vi "Create_Experiment_Excel_Files.vi"(1 "error in":errorcluster, 2 "Folder path in":path, 3 "Data in":T1={"User Name"="", "Experiment Number"=0, "Start Time"=timestamp(0 s since 1904-01-01), "Data"=[], "Step Number"=1, "Step Instructions"="", "Diagnostics"={"Langmuir Probe"=FALSE, "Rogowski 1"=FALSE, "Rogowski 2"=FALSE, "Rogowski 3"=FALSE, "B-dot 1"=FALSE, "B-dot 2"=FALSE}, "Experiment Purpose"="", "Experiment State"=enum."Off", "Systems"={"Compressed Air"=FALSE, "T-20kV Power Switch"=FALSE, "T-Rectifier"=FALSE, "Engage Interlock"=FALSE, "Ventilator"=FALSE, "Magnetron"=FALSE, "H-20kV Power Switch"=FALSE, "H-Rectifier"=FALSE, "Main Water Pump"=FALSE, "WEGA Water Pump"=FALSE, "Gas Inlet Valves"=FALSE}, "Vacuum Pressure"=0.0, "Fieldpoints"={"System Boolean Fieldpoints"={"Compressed Air"="", "T-20kV Power Switch"="", "T-Rectifier"="", "Engage Interlock"="", "Ventilator"="", "Magnetron"="", "H-20kV Power Switch"="", "H-Rectifier"="", "Main Water Pump"="", "WEGA Water Pump"="", "Gas Inlet Valves"=""}, "Step Fieldpoints"={"Exhaust Ventillator"="", "Compressed Air"="", "Water Pressure"="", "Interlock"="", "Toroidal Power Supply 1"="", "Toroidal Power Supply 2"="", "Toroidal Rectifier"="", "Helical Power Supply"="", "Helical Rectifier"="", "6kW Magnetron Standby"="", "20kW Magnetron Standby"=""}}, "Pressure History"={"Seconds into Experiment"=[], "Pressure Data"=[]}, "Time Computer Control"=[], "Toroidal Voltage Computer Control"=[], "Helical Voltage Computer Control"=[], "Toroidal Current"=[], "Toroidal Voltage"=[], "Toroidal Current Set Point"=[], "Helical Current Set Point"=[], "Helical Voltage"=[], "Helical Current"=[], "Experiment Folder"=path "", "Run Another Shot?"=FALSE}) -> (0 "error out":errorcluster)   [LabVIEW 2017]
uses:
  Type_Defs/Data.ctl
  Type_Defs/Diagnostics.ctl
  Type_Defs/Systems.ctl
  <vilib>/express/express shared/transition.llb/Dynamic To Waveform Array.vi
  <vilib>/express/express signal manip/GetorSetDDTAttributes/Set DDT Attributes/SetT0.vi
  <vilib>/express/express shared/transition.llb/Waveform Array To Dynamic.vi
  <vilib>/express/express signal manip/GetorSetDDTAttributes/Set DDT Attributes/Set DDT Properties.xnode
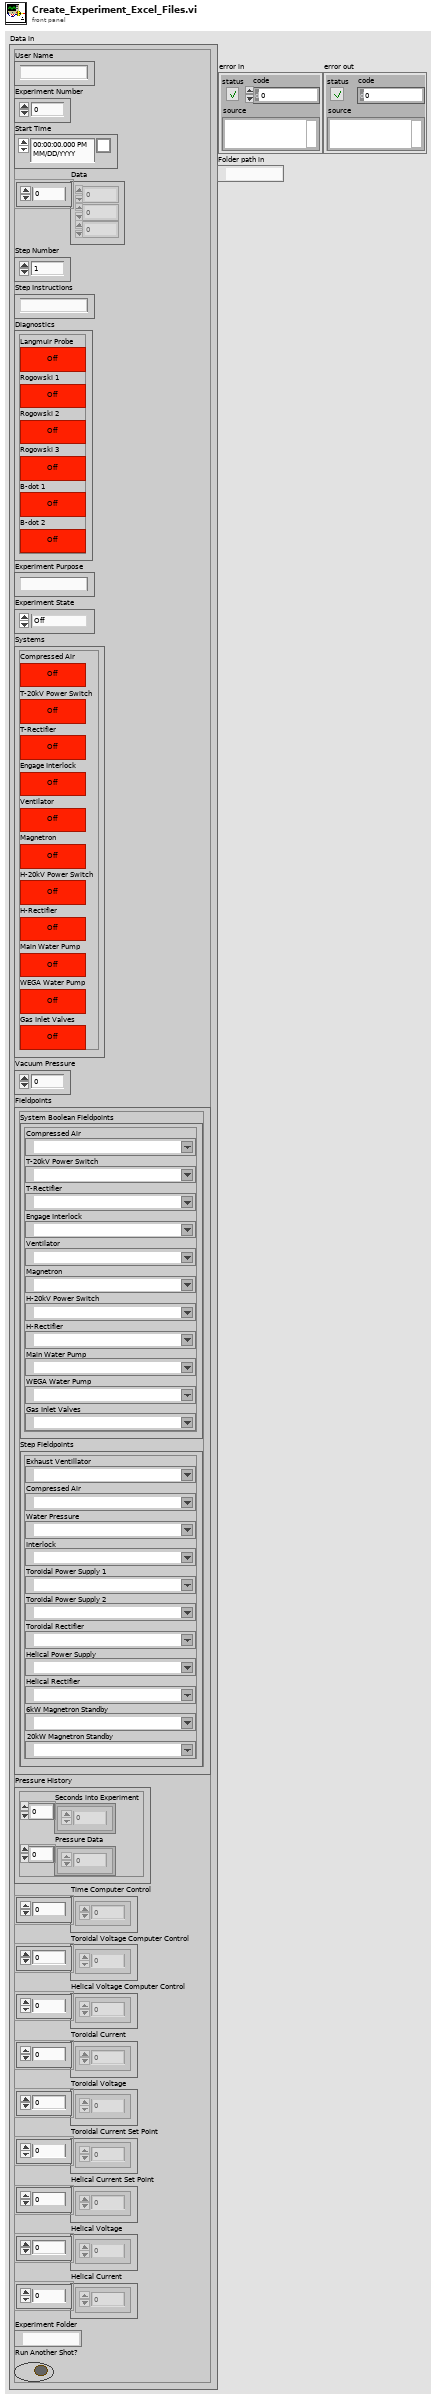
[diagram p1: front panel]
types:
  T1 = typedef "Data.ctl" = cluster{"User Name":string, "Experiment Number":i32, "Start Time":timestamp, "Data":dbl[], "Step Number":i32, "Step Instructions":string, "Diagnostics":T2, "Experiment Purpose":string, "Experiment State":enum16{"Off", "Setting Up", "Ready", "In Progress", "Shutting Down"}, "Systems":T3, "Vacuum Pressure":dbl, "Fieldpoints":cluster{"System Boolean Fieldpoints":cluster{"Compressed Air":refnum<k21>, "T-20kV Power Switch":refnum<k21>, "T-Rectifier":refnum<k21>, "Engage Interlock":refnum<k21>, "Ventilator":refnum<k21>, "Magnetron":refnum<k21>, "H-20kV Power Switch":refnum<k21>, "H-Rectifier":refnum<k21>, "Main Water Pump":refnum<k21>, "WEGA Water Pump":refnum<k21>, "Gas Inlet Valves":refnum<k21>}, "Step Fieldpoints":cluster{"Exhaust Ventillator":refnum<k21>, "Compressed Air":refnum<k21>, "Water Pressure":refnum<k21>, "Interlock":refnum<k21>, "Toroidal Power Supply 1":refnum<k21>, "Toroidal Power Supply 2":refnum<k21>, "Toroidal Rectifier":refnum<k21>, "Helical Power Supply":refnum<k21>, "Helical Rectifier":refnum<k21>, "6kW Magnetron Standby":refnum<k21>, "20kW Magnetron Standby":refnum<k21>}}, "Pressure History":cluster{"Seconds into Experiment":i32[], "Pressure Data":dbl[]}, "Time Computer Control":dbl[], "Toroidal Voltage Computer Control":dbl[], "Helical Voltage Computer Control":dbl[], "Toroidal Current":dbl[], "Toroidal Voltage":dbl[], "Toroidal Current Set Point":dbl[], "Helical Current Set Point":dbl[], "Helical Voltage":dbl[], "Helical Current":dbl[], "Experiment Folder":path, "Run Another Shot?":bool}
  T2 = typedef "Diagnostics.ctl" = cluster{"Langmuir Probe":bool, "Rogowski 1":bool, "Rogowski 2":bool, "Rogowski 3":bool, "B-dot 1":bool, "B-dot 2":bool}
  T3 = typedef "Systems.ctl" = cluster{"Compressed Air":bool, "T-20kV Power Switch":bool, "T-Rectifier":bool, "Engage Interlock":bool, "Ventilator":bool, "Magnetron":bool, "H-20kV Power Switch":bool, "H-Rectifier":bool, "Main Water Pump":bool, "WEGA Water Pump":bool, "Gas Inlet Valves":bool}
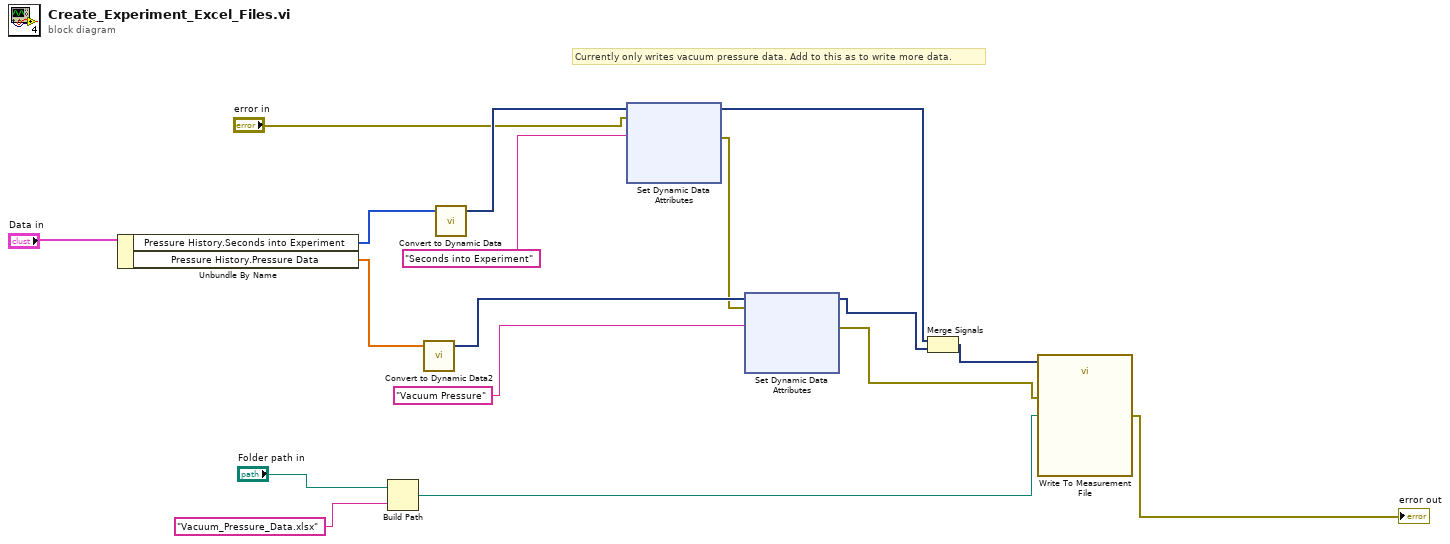
[diagram p0: block diagram]
diagram:
  # "Currently only writes vacuum pressure data. Add to this as to write more data."
  n1 = Unbundle By Name("Data in") -> ("Pressure History.Seconds into Experiment"=w2:i32[], "Pressure History.Pressure Data"=w1:dbl[])
  n2 = Build Path(base path="Folder path in", name or relative path="Vacuum_Pressure_Data.xlsx" ("string")) -> (appended path=w14:path)
  n3 = call "Convert to Dynamic Data2"("Array"=w1) -> ("Dynamic Data Type"=w10:dynamicdata)  [unwired: 3 in]
  n4 = call "Convert to Dynamic Data"("Array"=w2) -> ("Dynamic Data Type"=w8:dynamicdata)  [unwired: 3 in]
  n5 = xnode "Set Dynamic Data Attributes"("Signals In"=w8, "error in"="error in", "Signal Name"="Seconds into Experiment") -> ("Signals Out"=w5:dynamicdata, "error out"=w9:errorcluster)  [unwired: 1 in]
  n6 = xnode "Set Dynamic Data Attributes"("Signals In"=w10, "error in"=w9, "Signal Name"="Vacuum Pressure") -> ("Signals Out"=w6:dynamicdata, "error out"=w4:errorcluster)  [unwired: 1 in]
  n7 = Merge Signals(w5, w6) -> (w13:dynamicdata)
  n8 = call "Write To Measurement File"("Signals"=w13, "error in (no error)"=w4, "Filename"=w14) -> ("error out"=→"error out":errorcluster)  [unwired: 14 in, 2 out]
